vi "TargetHitCheck.vi"(5 "Y-Max":i32, 7 "Y-Min":i32, 8 "Start Y Speed":i32, 9 "Start X Speed":i32, 10 "X-Min":i32, 11 "X-Max":i32) -> (2 "Hit":bool, 3 "MaxHeight":i32)   [LabVIEW 2020, in "2021_17.lvclass"]
uses:
  2021_17.lvclass
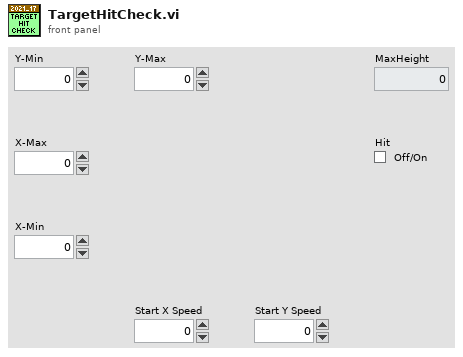
[diagram p1: front panel]
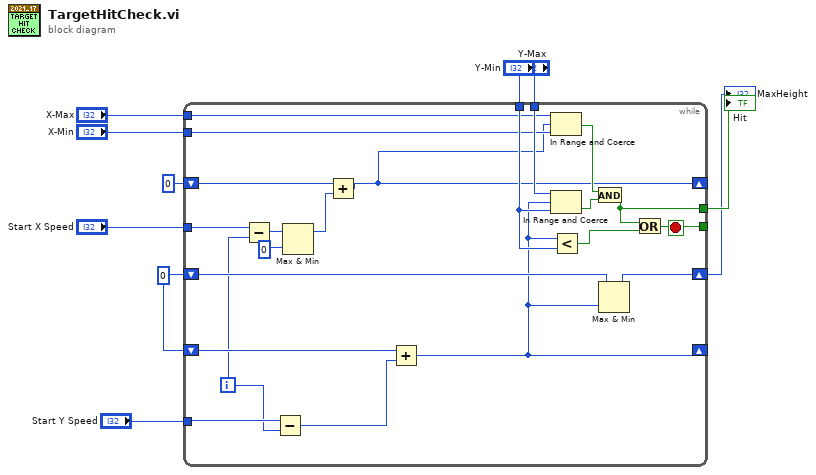
[diagram p0: block diagram]
diagram:
  w8 = 0
  n1 = while {
    tunnel: "Y-Max" -> [w32]
    tunnel: "Y-Min" -> [w31]
    tunnel: [w29] -> _
    tunnel: [w24] -> w10
    tunnel: "X-Max" -> [w28]
    tunnel: "X-Min" -> [w27]
    tunnel: "Start X Speed" -> [w20]
    shift-right: [w21] -> _
    shift-left: 0 -> [w22]
    shift-right: [w15] -> w7
    shift-left: w8 -> [w16]
    shift-right: [w11] -> _
    shift-left: w8 -> [w23]
    tunnel: "Start Y Speed" -> [w14]
    i -> [w13]
    stop <- w29 stop-if-true
    n2 = Subtract(x=w20, y=w13) -> (x-y=w19:i32)
    n3 = Subtract(x=w14, y=w13) -> (x-y=w12:i32)
    n4 = Max & Min(x=w19, y=0) -> (max(x,y)=w18:i32)  [unwired: 1 out]
    n5 = Add(x=w22, y=w18) -> (x+y=w21:i32)
    n6 = Add(x=w23, y=w12) -> (x+y=w11:i32)
    n7 = In Range and Coerce(upper limit=w28, x=w21, lower limit=w27) -> (In Range?=w25:bool)  [unwired: 1 out]
    n8 = In Range and Coerce(upper limit=w32, x=w11, lower limit=w31) -> (In Range?=w26:bool)  [unwired: 1 out]
    n9 = Less?(x=w11, y=w31) -> (x < y?=w30:bool)
    n10 = And(x=w25, y=w26) -> (x .and. y?=w24:bool)
    n11 = Max & Min(x=w16, y=w11) -> (max(x,y)=w15:i32)  [unwired: 1 out]
    n12 = Or(x=w24, y=w30) -> (x .or. y?=w29:bool)
  }
  "Hit" <- w10
  "MaxHeight" <- w7
